vi "Create_Table.vi"() -> (0 "String":string)   [LabVIEW 2011]
uses:
  Anemometry/Anemometry Sub Vis/Data_plotting_vis/Results_plotter_Global.vi
panel:
  out "Table Control":string[][](table)
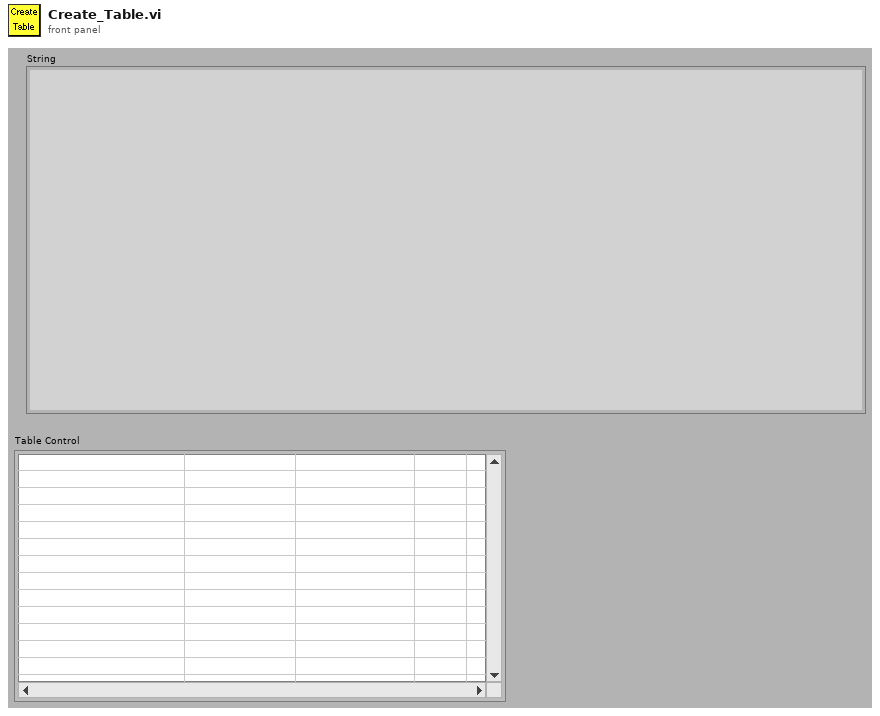
[diagram p1: front panel]
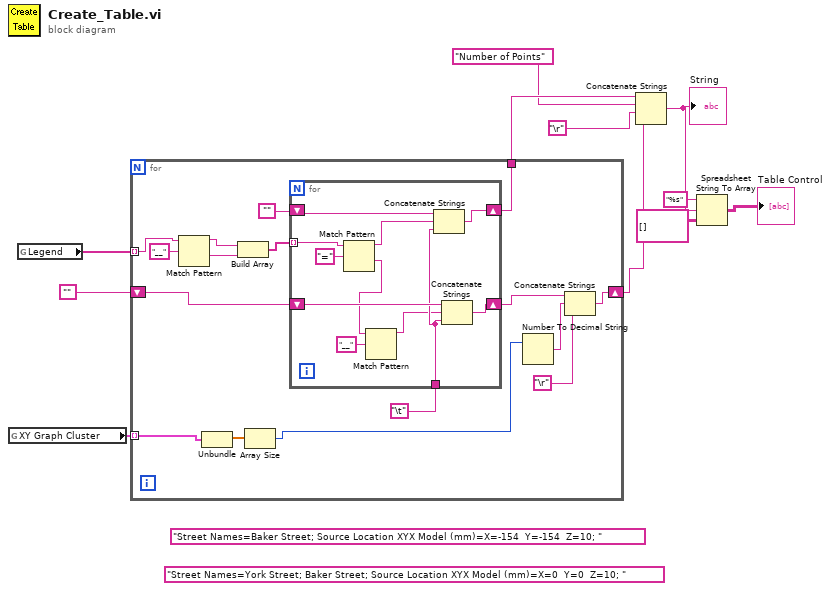
[diagram p0: block diagram]
diagram:
  (unwired) "Street Names=York Street; Baker Street; Source Location XYX Model (mm)=X=0  Y=0  Z=10; "
  (unwired) "Street Names=Baker Street; Source Location XYX Model (mm)=X=-154  Y=-154  Z=10; "
  n1 = global read "Results_plotter_Global.vi" "XY Graph Cluster"() -> (w10:cluster{dbl[], dbl[]}[])
  n2 = global read "Results_plotter_Global.vi" "Legend"() -> (w11:string[])
  n3 = for {
    tunnel: w11 -> [w15] mode=indexing
    tunnel: w10 -> [w27] mode=indexing
    shift-right: [w19] -> w5
    shift-left: "" -> [w25]
    tunnel: [w17] -> w8
    n4 = Match Pattern(string=w15, regular expression="__") -> (before substring=w14:string, after substring=w13:string)  [unwired: 1 in, 2 out]
    n5 = Unbundle(w27) -> (w26:dbl[])  [unwired: 1 out]
    n6 = Build Array(w14, w13) -> (w12:string[])
    n7 = Array Size(array=w26) -> (size(s)=w23:i32)
    n8 = for {
      tunnel: w12 -> [w37] mode=indexing
      shift-right: [w35] -> w22
      shift-left: w25 -> [w36]
      tunnel: "\t" -> [w32]
      shift-right: [w34] -> w17
      shift-left: "" -> [w33]
      n9 = Match Pattern(string=w37, regular expression="=") -> (before substring=w31:string, after substring=w29:string)  [unwired: 1 in, 2 out]
      n10 = Match Pattern(string=w29, regular expression="__") -> (before substring=w28:string)  [unwired: 1 in, 3 out]
      n11 = Concatenate Strings(w33, w31, w32) -> (w34:string)
      n12 = Concatenate Strings(w36, w28, w32) -> (w35:string)
    }
    n13 = Number To Decimal String(number=w23) -> (decimal integer string=w21:string)  [unwired: 1 in]
    n14 = Concatenate Strings(w22, w21, "\r") -> (w19:string)
  }
  n15 = Concatenate Strings(w8, "Number of Points" ("string"), "\r", w5) -> (w4:string)
  "String" <- w4
  n16 = Spreadsheet String To Array(format string="%s", spreadsheet string=w4, array type (2D Dbl)=string[][] []) -> (array=→"Table Control":string[][])  [unwired: 1 in]
